vi "Read Custom Header Info.vi"(8 "error in (no error)":errorcluster, 11 "Node Ptr":T1 format="%.0x") -> (0 "error out":errorcluster, 1 "CustomHeaderEnabled":bool, 2 "CustomHeaderLogicProfile":string, 3 "Node Ptr out":T1 format="%.0x")   [LabVIEW 2019, in "UDP-Custom-Device System Explorer.lvlib" / "Shared Packet Accessors.lvlib"]
uses:
  Shared Packet Accessors.lvlib
  <vilib>/NI VeriStand/Custom Device API/Custom Device Item Ref.ctl
  Shared/Constants.vi
  <vilib>/NI VeriStand/Custom Device API/Get Item Property (Boolean).vi
  <vilib>/NI VeriStand/Custom Device API/Get Item Property (String).vi
  <vilib>/NI VeriStand/Custom Device API/Custom Device API.lvlib
  Shared/UDP-Custom-Device Shared.lvlib
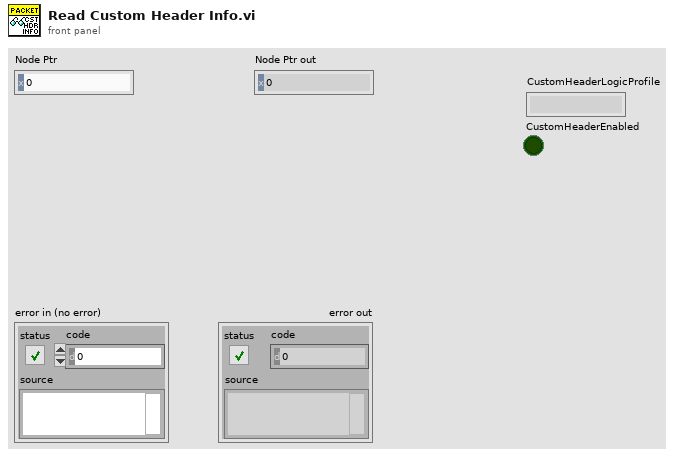
[diagram p1: front panel]
types:
  T1 = typedef "Custom Device API.lvlib/Custom Device Item Ref.ctl" = u64
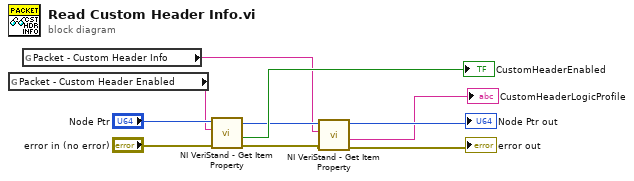
[diagram p0: block diagram]
diagram:
  n1 = global read "Constants.vi" "Packet - Custom Header Enabled"() -> (w8:string)
  n2 = global read "Constants.vi" "Packet - Custom Header Info"() -> (w2:string)
  n3 = call-poly <vilib>:"NI VeriStand - Get Item Property.vi"("error in (no error)"="error in (no error)", "Property Name"=w8, "Item Ref in"="Node Ptr") -> ("error out"=w6:errorcluster, "Value"=→"CustomHeaderEnabled":bool, "Item Ref out"=w4:T1)  [unwired: 5 in, 1 out]
  n4 = call-poly <vilib>:"NI VeriStand - Get Item Property.vi"("error in (no error)"=w6, "Property Name"=w2, "Item Ref in"=w4) -> ("error out"=→"error out":errorcluster, "Value"=→"CustomHeaderLogicProfile":string, "Item Ref out"=→"Node Ptr out":T1)  [unwired: 5 in, 1 out]
